vi "NodMcu interlink labview_2.vi"() -> ()   [LabVIEW 2015]
panel:
  out "Voltage":string
  in  "stop":bool
  out "Voltage(0-3.3v)":dbl(graph)
  in  "address":string
  # "Pardeep Kumar"
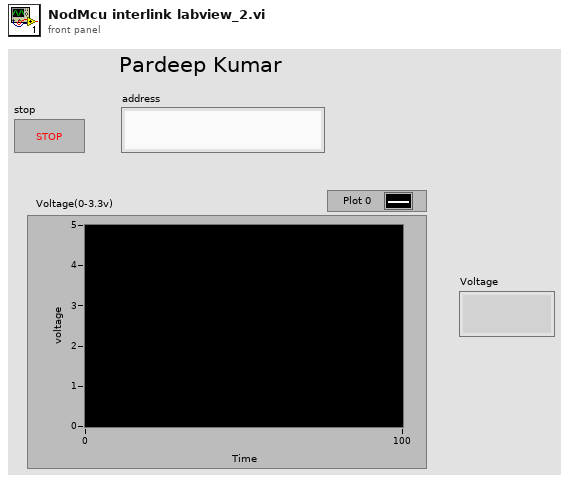
[diagram p1: front panel]
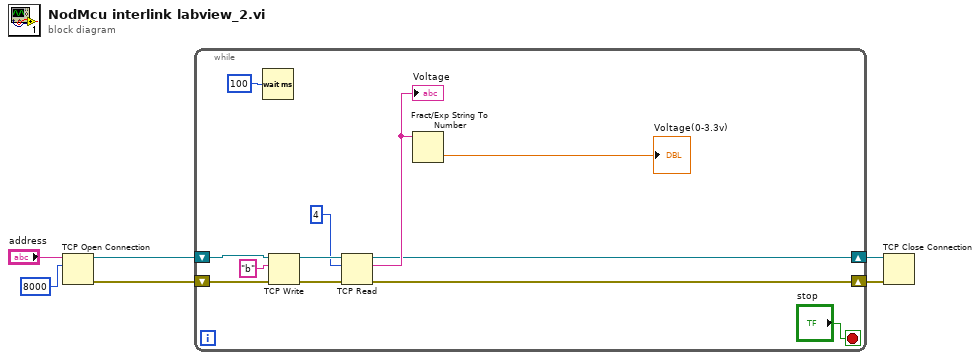
[diagram p0: block diagram]
diagram:
  n1 = TCP Open Connection(address="address", remote port or service name=u16 8000) -> (connection ID=w4:refnum<k5>, error out=w3:errorcluster)  [unwired: 3 in]
  n2 = while {
    shift-right: [w8] -> w2
    shift-left: w4 -> [w18]
    shift-right: [w7] -> w1
    shift-left: w3 -> [w17]
    stop <- "stop" stop-if-true
    n3 = Wait (ms)(milliseconds to wait=u32 100) -> ()  [unwired: 1 out]
    n4 = TCP Write(connection ID=w18, data in="b", error in (no error)=w17) -> (connection ID out=w16:refnum<k5>, error out=w15:errorcluster)  [unwired: 1 in, 1 out]
    n5 = TCP Read(connection ID=w16, bytes to read=4, error in (no error)=w15) -> (connection ID out=w8:refnum<k5>, data out=w11:string, error out=w7:errorcluster)  [unwired: 2 in]
    "Voltage" <- w11
    n6 = Fract/Exp String To Number(string=w11) -> (number=→"Voltage(0-3.3v)":dbl)  [unwired: 3 in, 1 out]
  }
  n7 = TCP Close Connection(connection ID=w2, error in (no error)=w1) -> ()  [unwired: 1 in, 2 out]
